vi "Reverse-Factorials.vi"() -> ()   [LabVIEW 2014]
panel:
  out "isFactorial?":string
  in  "Input":i32
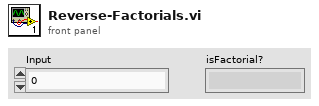
[diagram p1: front panel]
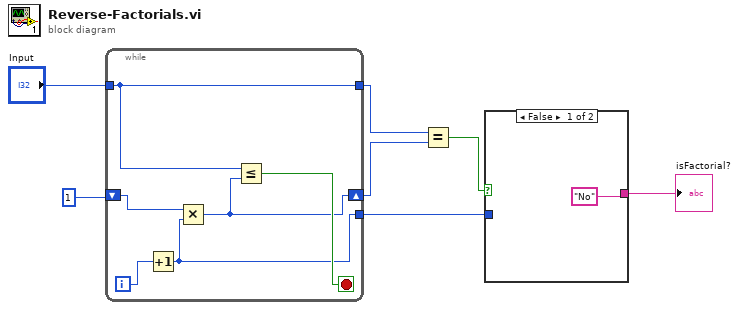
[diagram p0: block diagram]
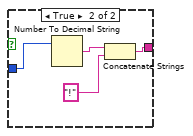
[diagram p2: hidden frame]
diagram:
  n1 = while {
    tunnel: "Input" -> [w11]
    shift-right: [w10] -> w5
    shift-left: 1 -> [w13]
    tunnel: [w11] -> w6
    tunnel: [w8] -> w3
    i -> [w9]
    stop <- w12 stop-if-true
    n2 = Increment(x=w9) -> (x+1=w8:i32)
    n3 = Multiply(x=w13, y=w8) -> (x*y=w10:i32)
    n4 = Less Or Equal?(x=w11, y=w10) -> (x <= y?=w12:bool)
  }
  n5 = Equal?(x=w6, y=w5) -> (x = y?=w4:bool)
  n6 = case shown="False" w4 {
    tunnel: w3 -> [_ w18]
    tunnel: ["No" w15] -> w2
    frame False {
    }
    frame True {
      n7 = Number To Decimal String(number=w18) -> (decimal integer string=w17:string)  [unwired: 1 in]
      n8 = Concatenate Strings(w17, "!") -> (w15:string)
    }
  }
  "isFactorial?" <- w2
